vi "CACH_0@7.vi"(6 "err in":errorcluster, 8 "Pu":dbl, 9 "Qa":dbl) -> (0 "err out":errorcluster, 3 "Cach":dbl)   [LabVIEW 2010, in "lv_07.lvlib"]
doc: "Calcul du prix d'achat (Annuel) Cach= Qa * Pu \nQa : Qté annuelle consommée\nPu : Prix unitaire Hors taxes de la pièce"
uses:
  lv_07.lvlib
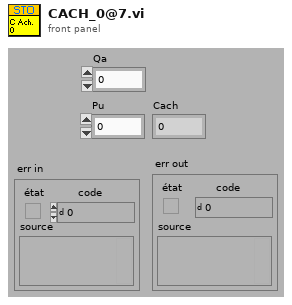
[diagram p1: front panel]
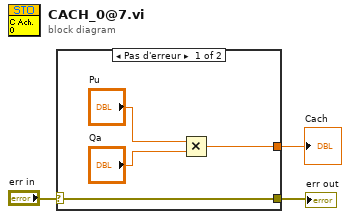
[diagram p0: block diagram]
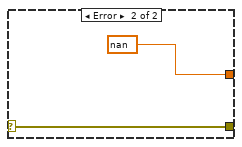
[diagram p2: hidden frame]
diagram:
  n1 = case shown="Pas d'erreur" "err in" {
    selector: "err in" -> [w5 w9]
    tunnel: [w5 w9] -> w2
    tunnel: [w4 nan] -> w1
    frame No Error {
      n2 = Multiply(x="Pu", y="Qa") -> (x*y=w4:dbl)
    }
    frame Error {
    }
  }
  "err out" <- w2
  "Cach" <- w1
